vi "Errors.vi"   [LabVIEW 2017, in "DSF Core.lvlib" / "DSF PXImc Transceiver.lvclass"]
uses:
  DSF PXImc Transceiver.lvclass
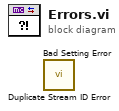
[diagram p0: block diagram]
diagram:
  n1 = call "Duplicate Stream ID Error.vi"() -> ()  [unwired: 10 in, 2 out]
  n2 = call "Bad Setting Error.vi"() -> ()  [unwired: 10 in, 2 out]
